vi "VI Tree.vi"   [LabVIEW 2018, in "Agilent U2722.lvlib"]
doc: "This is the instrument driver for the Agilent U2722A and U2723A USB Modular Source Measure Unit. The VI Tree displays all the user-callable VIs of the instrument driver in an organized table."
uses:
  Agilent U2722.lvlib
  Configure/Configure Channel (Current).vi
  Data/Read Output (Single).vi
panel:
  # "(c) 2009-2015 National Instruments.  ALL RIGHTS RESERVED."
  # "SEE DIAGRAM\nFOR VI TREE."
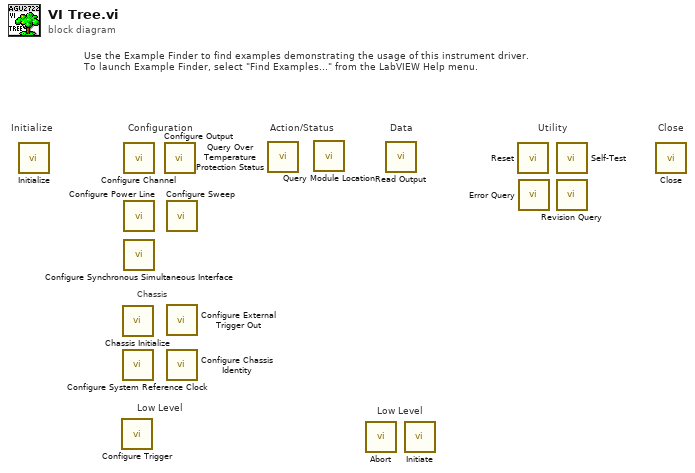
[diagram p0: block diagram]
diagram:
  # "Low Level"
  # "Chassis"
  # "Low Level"
  # "Use the Example Finder to find examples demonstrating the usage of this instrument driver.\nTo launch Example Finder, select \"Find Examples...\" from the LabVIEW Help menu."
  # "Configuration"
  # "Utility"
  # "Data"
  # "Action/Status"
  # "Close"
  # "Initialize"
  n1 = call <instrlib>:"Initialize.vi"() -> ()  [unwired: 10 in, 2 out]
  n2 = call "Configure Trigger.vi"() -> ()  [unwired: 10 in, 2 out]
  n3 = call "Chassis Initialize.vi"() -> ()  [unwired: 10 in, 2 out]
  n4 = call "Configure System Reference Clock.vi"() -> ()  [unwired: 10 in, 2 out]
  n5 = call-poly "Configure Channel.vi"() -> ()  [unwired: 10 in, 2 out]
  n6 = call <instrlib>:"Configure Power Line.vi"() -> ()  [unwired: 10 in, 2 out]
  n7 = call "Configure Synchronous Simultaneous Interface.vi"() -> ()  [unwired: 10 in, 2 out]
  n8 = call "Configure Output.vi"() -> ()  [unwired: 10 in, 2 out]
  n9 = call <instrlib>:"Configure Sweep.vi"() -> ()  [unwired: 10 in, 2 out]
  n10 = call "Configure External Trigger Out.vi"() -> ()  [unwired: 10 in, 2 out]
  n11 = call "Configure Chassis Identity.vi"() -> ()  [unwired: 10 in, 2 out]
  n12 = call "Query Over Temperature Protection Status.vi"() -> ()  [unwired: 9 in, 3 out]
  n13 = call "Query Module Location.vi"() -> ()  [unwired: 8 in, 4 out]
  n14 = call "Abort.vi"() -> ()  [unwired: 10 in, 2 out]
  n15 = call-poly "Read Output.vi"() -> ()  [unwired: 8 in, 4 out]
  n16 = call "Initiate.vi"() -> ()  [unwired: 10 in, 2 out]
  n17 = call <instrlib>:"Reset.vi"() -> ()  [unwired: 10 in, 2 out]
  n18 = call "Error Query.vi"() -> ()  [unwired: 8 in, 4 out]
  n19 = call "Self-Test.vi"() -> ()  [unwired: 8 in, 4 out]
  n20 = call "Revision Query.vi"() -> ()  [unwired: 8 in, 4 out]
  n21 = call <instrlib>:"Close.vi"() -> ()  [unwired: 11 in, 1 out]
